vi "Set Timing Information.vi"(8 "error in (no error)":errorcluster, 9 "offset":i32, 10 "decimation":i32, 11 "DSFTiming in":refnum<class "DSFTiming.lvclass">) -> (0 "error out":errorcluster, 3 "DSFTiming out":refnum<class "DSFTiming.lvclass">)   [LabVIEW 2017, in "DSFTiming.lvclass"]
uses:
  DSFTiming.lvclass
  DSFTiming.lvclass/DSFTiming.ctl
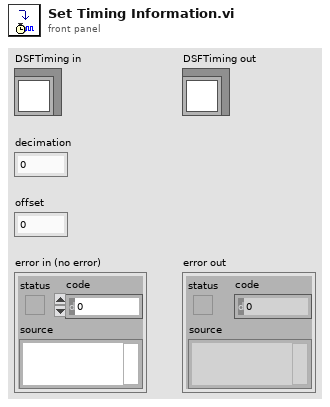
[diagram p1: front panel]
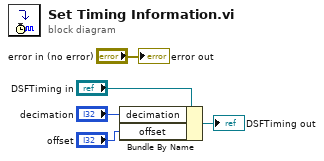
[diagram p0: block diagram]
diagram:
  n1 = Bundle By Name(cluster="DSFTiming in", "decimation"="decimation", "offset"="offset") -> (→"DSFTiming out":refnum<class "DSFTiming.lvclass">)
  "error out" <- "error in (no error)"
